vi "Teleop.vi"(10 "Match Info":T1={"Autonomous Elapsed Seconds"=0.0, "TeleOp Elapsed Seconds"=0.0, "Disabled Elapsed Seconds"=0.0, "Visited Autonomous"=FALSE, "Visited TeleOp"=FALSE, "Visited Disabled"=FALSE, "Autonomous Settings"={"Autonomous Style"=enum."Independent", "VI Refnum"=refnum}}, 11 "Call Context":T2) -> ()   [LabVIEW 2016]
doc: "This VI is called for each TeleOp packet received from the DS where the robot is not disabled. It is often used to read from the joysticks and update I/O or to update setpoints for timed control loops. It should complete and return within 20 milliseconds or it may miss DS packets."
uses:
  <vilib>/Rock Robotics/WPI/DriverStation/WPI_DriverStationDerivedRobotMode.ctl
  <vilib>/Rock Robotics/WPI/DriverStation/WPI_DriverStationMatch Info.ctl
  <vilib>/Rock Robotics/WPI/Utilities/WPI_GetSetVariantRefNum.vi
  <vilib>/Rock Robotics/WPI/Ultrasonic/WPI_SonarMB1010DigitalRefNum Registry Get.vi
  <vilib>/Rock Robotics/WPI/Ultrasonic/WPI_SonarMB1010DigitalGetRange.vi
  FRC SimulatedRSC/Positions.vi
panel:
  in  "Set RPM":dbl=7000.0 format="%#_13g"
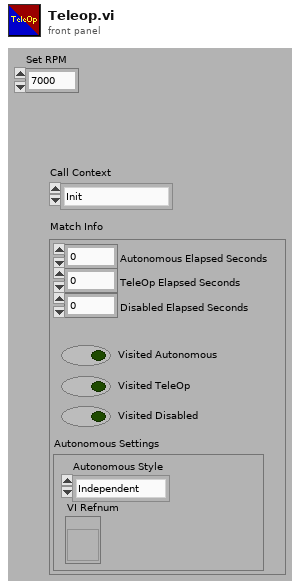
[diagram p1: front panel]
types:
  T1 = typedef "WPI_DriverStationMatch Info.ctl" = cluster{"Autonomous Elapsed Seconds":dbl, "TeleOp Elapsed Seconds":dbl, "Disabled Elapsed Seconds":dbl, "Visited Autonomous":bool, "Visited TeleOp":bool, "Visited Disabled":bool, "Autonomous Settings":cluster{"Autonomous Style":enum16{"Iterative", "Independent"}, "VI Refnum":refnum<vi>}}
  T2 = typedef "WPI_DriverStationDerivedRobotMode.ctl" = enum16{"Init", "Execute", "Stop"}
  T3 = typedef "WPI_JoystickDevRef.ctl" = cluster{"Device":T4}
  T4 = typedef "WPI_JoystickDeviceEnum.ctl" = enum16{"USB 0", "USB 1", "USB 2", "USB 3", "USB 4", "USB 5"}
  T5 = typedef "WPI_SonarMB1010DigitalDeviceRef.ctl" = cluster{"CounterDevRef":T6, "Scaling factor (s/in)":dbl}
  T6 = typedef "WPI_CounterDevRef.ctl" = cluster{"DevStatus":errorcluster, "CntIndex":T7}
  T7 = typedef "FPGA_CounterCtrSystemIndex.ctl" = enum8{"Ctr 0", "Ctr 1", "Ctr 2", "Ctr 3", "Ctr 4", "Ctr 5", "Ctr 6", "Ctr 7", "Invalid"}
  T8 = typedef "WPI_MotorControlDeviceRef.ctl" = cluster{"DeviceStatus":errorcluster, "Type":T9, "PWM":cluster{"PWM Channel":T10, "DeadBand":T11}, "CAN":cluster{"Device Number":u8, "SetOutput VI Ref":variant, "GetOutput VI Ref":variant, "Enable VI Ref":variant, "Disable VI Ref":variant, "Data":variant}, "Invert":bool}
  T9 = typedef "WPI_MotorControlType.ctl" = enum16{"PWM", "CAN"}
  T10 = typedef "FPGA_DIOPWMChannel.ctl" = enum8{"PWM 0", "PWM 1", "PWM 2", "PWM 3", "PWM 4", "PWM 5", "PWM 6", "PWM 7", "PWM 8", "PWM 9", "PWM MXP 0", "PWM MXP 1", "PWM MXP 2", "PWM MXP 3", "PWM MXP 4", "PWM MXP 5", "PWM MXP 6", "PWM MXP 7", "PWM MXP 8", "PWM MXP 9", "Invalid"}
  T11 = typedef "WPI_PWMDeadband.ctl" = cluster{"Name":string, "maxPositivePwm":i32, "minPositivePwm":i32, "centerPwm":i32, "maxNegativePwm":i32, "minNegativePwm":i32, "angularRange":u16}
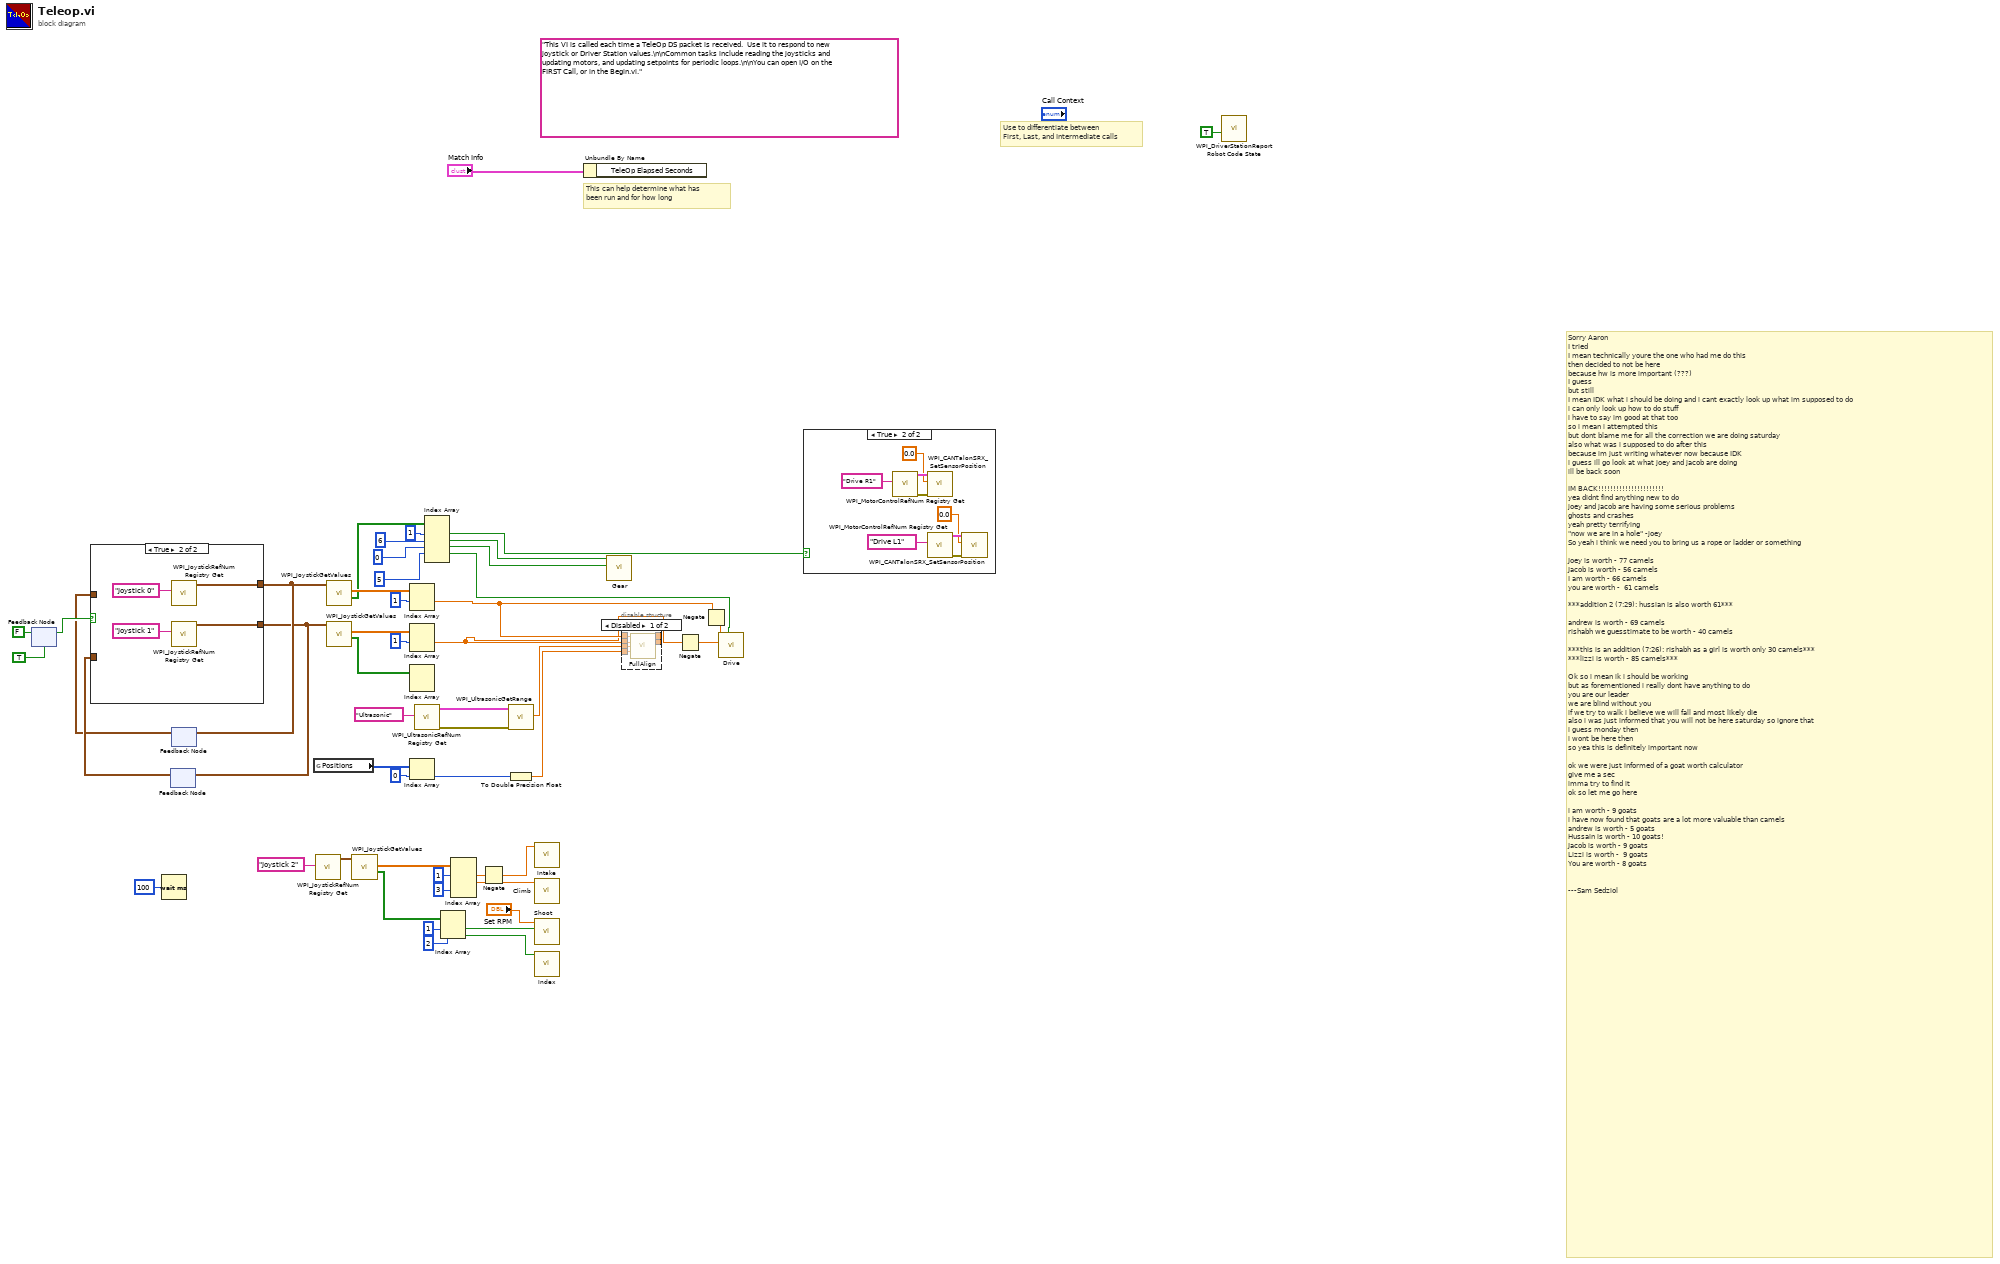
[diagram p0: block diagram]
diagram:
  (unwired) "This VI is called each time a TeleOp DS packet is received.  Use it to respond to new joystick or Driver Station values.\n\nCommon tasks include reading the joysticks and updating motors, and updating setpoints for periodic loops.\n\nYou can open I/O on the FIRST Call, or in the Begin.vi."
  # "Sorry Aaron\nI tried\nI mean technically youre the one who had me do this\nthen decided to not be here\nbecause hw is more important (???)\nI guess\nbut still\nI mean IDK what i should be doing and i cant exactly look up what im supposed to do\ni can only look up how to do stuff\ni have to say im good at that too\nso i mean i attempted this\nbut dont blame me for all the correction we are doing saturday\nalso what was i supposed to do after this\nbecause im just writing whatever now because IDK\ni guess ill go look at what joey and jacob are doing\nill be back soon\n\nIM BACK!!!!!!!!!!!!!!!!!!!!!!\nyea didnt find anything new to do\njoey and jacob are having some serious problems\nghosts and crashes\nyeah pretty terrifying\n\"now we are in a hole\" -joey\nSo yeah i think we need you to bring us a rope or ladder or something\n\nJoey is worth - 77 camels\nJacob is worth - 56 camels\nI am worth - 66 camels\nyou are worth -  61 camels \n\n***addition 2 (7:29): hussian is also worth 61***\n\nandrew is worth - 69 camels\nrishabh we guesstimate to be worth - 40 camels\n\n***this is an addition (7:26): rishabh as a girl is worth only 30 camels***\n***lizzi is worth - 85 camels***\n\nOk so i mean ik i should be working\nbut as forementioned i really dont have anything to do\nyou are our leader\nwe are blind without you\nif we try to walk i believe we will fall and most likely die\nalso i was just informed that you will not be here saturday so ignore that\ni guess monday then\ni wont be here then\nso yea this is definitely important now\n\nok we were just informed of a goat worth calculator\ngive me a sec \nimma try to find it\nok so let me go here\n\ni am worth - 9 goats\ni have now found that goats are a lot more valuable than camels\nandrew is worth - 5 goats\nHussain is worth - 10 goats! \nJacob is worth - 9 goats\nLizzi is worth -  9 goats\nYou are worth - 8 goats\n\n\n---Sam Sedziol"
  # "Use to differentiate between\nFirst, Last, and Intermediate calls"
  # "This can help determine what has\nbeen run and for how long"
  n1 = feedback-in #1(FALSE) -> ()
  n2 = feedback #1(TRUE) -> (w20:bool)
  n3 = Wait (ms)(milliseconds to wait=u32 100) -> ()  [unwired: 1 out]
  n4 = feedback #2() -> (w16:T3)  [unwired: 1 in]
  n5 = feedback #3() -> (w15:T3)  [unwired: 1 in]
  n6 = case shown="True" w20 {
    tunnel: [w52 w56] -> w18
    tunnel: [w51 w55] -> w17
    tunnel: w16 -> [w51 _]
    tunnel: w15 -> [w52 _]
    frame False {
    }
    frame True {
      n7 = call <vilib>:"WPI_JoystickRefNum Registry Get.vi"("refnum name"="Joystick 0") -> ("JoystickDevRef"=w56:T3)  [unwired: 1 in, 9 out]
      n8 = call <vilib>:"WPI_JoystickRefNum Registry Get.vi"("refnum name"="Joystick 1") -> ("JoystickDevRef"=w55:T3)  [unwired: 1 in, 9 out]
    }
  }
  n9 = feedback-in #2(w17) -> ()
  n10 = feedback-in #3(w18) -> ()
  n11 = global read "Positions.vi" "Positions"() -> (w23:i32[])
  n12 = call <vilib>:"WPI_JoystickRefNum Registry Get.vi"("refnum name"="Joystick 2") -> ("JoystickDevRef"=w45:T3)  [unwired: 1 in, 9 out]
  n13 = call <vilib>:"WPI_JoystickGetValues.vi"("JoystickDevRef"=w18) -> ("Buttons"=w41:bool[], "Axes"=w48:dbl[])  [unwired: 6 in, 3 out]
  n14 = call <vilib>:"WPI_JoystickGetValues.vi"("JoystickDevRef"=w17) -> ("Buttons"=w42:bool[], "Axes"=w47:dbl[])  [unwired: 6 in, 3 out]
  n15 = call <vilib>:"WPI_JoystickGetValues.vi"("JoystickDevRef"=w45) -> ("Buttons"=w43:bool[], "Axes"=w44:dbl[])  [unwired: 6 in, 3 out]
  n16 = Index Array(array=w48, index #1=1 ("index")) -> (element #1=w25:dbl)  [unwired: 1 in, 1 out]
  n17 = Index Array(array=w47, index #1=1 ("index")) -> (element #1=w24:dbl)  [unwired: 1 in, 1 out]
  n18 = Index Array(array=w42) -> ()  [unwired: 2 in, 2 out]
  n19 = Index Array(array=w23, index=0) -> (element=w30:i32)
  n20 = call-poly <vilib>:"WPI_UltrasonicRefNum Registry Get.vi"("refnum name"="Ultrasonic") -> ("error out"=w36:errorcluster, "SonarMB1010DigitalDevRef"=w37:T5)  [unwired: 9 in]
  n21 = Index Array(array=w41, index #1=1 ("index"), index #2=6 ("index"), index #3=0 ("index"), index #4=5 ("index")) -> (element #1=w33:bool, element #2=w5:bool, element #3=w4:bool, element #4=w1:bool)  [unwired: 1 in, 1 out]
  n22 = Index Array(array=w43, index #1=1 ("index"), index #2=2 ("index")) -> (element #1=w27:bool, element #2=w26:bool)
  n23 = Index Array(array=w44, index #1=1 ("index"), index #2=3 ("index")) -> (element #1=w38:dbl, element #2=w28:dbl)  [unwired: 2 in, 2 out]
  n24 = Negate(x=w38) -> (-x=w10:dbl)
  n25 = call-poly <vilib>:"WPI_UltrasonicGetRange.vi"("error in"=w36, "SonarMB1010DigitalDevRef"=w37) -> ("Distance"=w34:dbl)  [unwired: 7 in, 2 out]
  n26 = To Double Precision Float(number=w30) -> (double precision float=w29:dbl)
  n27 = call "Intake.vi"("Effort"=w10) -> ()  [unwired: 11 in]
  n28 = call "Climb.vi"("Effort"=w28) -> ()  [unwired: 11 in]
  n29 = call "Shoot.vi"("Shoot?"=w27, "Set RPM"="Set RPM") -> ()  [unwired: 10 in]
  n30 = call "Index.vi"("Index?"=w26) -> ()  [unwired: 11 in]
  n31 = Unbundle By Name("Match Info") -> ()  [unwired: 1 out]
  n32 = call "Gear.vi"("Gear1?"=w4, "Gear0?"=w5) -> ()  [unwired: 10 in]
  n33 = disable-structure shown="Disabled" {
    disable-tunnel: w25 -> [w62 _]
    disable-tunnel: w24 -> [w61 _]
    disable-tunnel: w34 -> [w60 _]
    disable-tunnel: w29 -> [w59 _]
    disable-tunnel: [w58 _] -> _
    disable-tunnel: [w57 _] -> _
    frame Disabled {
      n34 = call "FullAlign.vi"("Joystick 0"=w62, "Joystick 1"=w61, "Distance"=w60, "Angle"=w59) -> ("Right Motor"=w57:dbl, "Left Motor"=w58:dbl)  [unwired: 9 in, 1 out]
    }
    frame Enabled {
    }
  }
  n35 = Negate(x=w24) -> (-x=w6:dbl)
  n36 = Negate(x=w25) -> (-x=w7:dbl)
  n37 = call "Drive.vi"("Slow?"=w1, "Drive L"=w6, "Drive R"=w7) -> ()  [unwired: 9 in]
  n38 = case shown="True" w33 {
    frame False {
    }
    frame True {
      n39 = call <vilib>:"WPI_MotorControlRefNum Registry Get.vi"("refnum name"="Drive R1") -> ("error out"=w65:errorcluster, "MotorControlDevRef"=w64:T8)  [unwired: 9 in]
      n40 = call <vilib>:"WPI_CANTalonSRX_SetSensorPosition.vi"("error in (no error)"=w65, "New Sensor Position"=0.0, "CAN Talon SRX Ref"=w64) -> ()  [unwired: 7 in, 2 out]
      n41 = call <vilib>:"WPI_MotorControlRefNum Registry Get.vi"("refnum name"="Drive L1") -> ("error out"=w67:errorcluster, "MotorControlDevRef"=w68:T8)  [unwired: 9 in]
      n42 = call <vilib>:"WPI_CANTalonSRX_SetSensorPosition.vi"("error in (no error)"=w67, "New Sensor Position"=0.0, "CAN Talon SRX Ref"=w68) -> ()  [unwired: 7 in, 2 out]
    }
  }
  n43 = call <vilib>:"WPI_DriverStationReport Robot Code State.vi"("TeleOp"=TRUE ("Autonomous")) -> ()  [unwired: 10 in, 1 out]
